vi "_rszvl_core_repcap_channel.vi"(1 "Channel":i32) -> (0 "Rep cap":string)   [LabVIEW 2014]
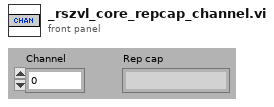
[diagram p1: front panel]
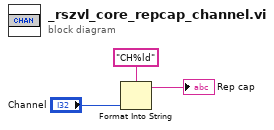
[diagram p0: block diagram]
diagram:
  n1 = Format Into String(format string="CH%ld", "Channel") -> (resulting string=→"Rep cap":string)  [unwired: 2 in, 1 out]
